vi "main.vi"() -> ()   [LabVIEW 2021]
uses:
  <vilib>/Analysis/Matrix/Datatypes/RealMatrix.ctl
  <vilib>/myRIO/Common/Instrument Driver Framework/myRIO v1.0/IRQ/typedefs/DI IRQ Type.ctl
  <vilib>/userDefined/High Color/nirio_resource_hc.ctl
  <vilib>/myRIO/Instrument Drivers/Onboard IO/PWM/typedefs/PWM Reference.ctl
  <vilib>/myRIO/Common/Instrument Driver Framework/Utilities/typedefs/myRIO Generic Hardware Reference.ctl
  <vilib>/myRIO/Common/Instrument Driver Framework/Utilities/typedefs/Hardware Version Enum.ctl
  <vilib>/myRIO/Common/Instrument Driver Framework/Utilities/typedefs/myRIO v1.0 Reference.ctl
  <vilib>/myRIO/Common/Instrument Driver Framework/Utilities/typedefs/Generic FPGA Reference.ctl
  <vilib>/myRIO/Common/Instrument Driver Framework/myRIO v1.0/PWM/typedefs/PWM Channels Enum.ctl
  <vilib>/myRIO/Instrument Drivers/Onboard IO/PWM/typedefs/PWM Configuration.ctl
  <vilib>/Platform/TimedLoop/XDataNode/timing_clust.ctl
  <vilib>/Platform/TimedLoop/XDataNode/nitl_modes.ctl
  <vilib>/Platform/TimedLoop/XDataNode/wakeup.ctl
  <vilib>/myRIO/Instrument Drivers/Onboard IO/PWM/vis/Set Duty Cycle and Frequency.vi
  ISRglobals.vi
  ISR.vi
  <vilib>/myRIO/Common/Instrument Driver Framework/myRIO v1.0/IRQ/vis/myRIO v1.1 Register DI IRQ.vi
  <vilib>/Analysis/Matrix/Numeric/Multiply/Multiply - RM,R.vi
  <vilib>/Analysis/Matrix/Numeric/Multiply/Multiply - RM,RM.vi
  <vilib>/myRIO/Common/Instrument Driver Framework/myRIO v1.0/PWM/vis/myRIO v1.0 Write PWM.vi
  <vilib>/myRIO/Express VI/IRQ/IRQ Express VI.xnode
  <vilib>/myRIO/Instrument Drivers/IRQ/IO IRQ/vis/myRIO Register DI IRQ.xnode
  <vilib>/myRIO/Common/Instrument Driver Framework/myRIO v1.0/IRQ/typedefs/Callback VI Ref.ctl
  <vilib>/platform/TimedLoop/XDataNode/XDataNode.xnode
  <vilib>/Platform/TimedLoop/XDataNode/XDNodeRunTimeDep.lvlib
  <vilib>/myRIO/Instrument Drivers/Onboard IO/PWM/PWM.lvlib
  <vilib>/Analysis/Matrix/NI_Matrix.lvlib
  <vilib>/ptbypt/NI_PtbyPt.lvlib
panel:
  out "theta RLS":dbl[][](graph)
  out "theta_RLS_1":dbl[](graph)
  out "theta_RLS_0":dbl[](graph)
  out "theta_RLS_2":dbl[](graph)
  out "theta_RLS_3":dbl[](graph)
  out "theta 3":dbl[](graph)
  out "theta 2":dbl[](graph)
  out "theta 1":dbl[](graph)
  out "theta 0":dbl[](graph)
  out "u":dbl
  out "PWM":dbl
  out "up":dbl
  out "uw":dbl
  out "Omega_d":dbl[][](graph)
  out "theta":dbl[][](graph)
  out "U":dbl[][](graph)
  out "th_max":T1
  out "th_min":T1
  out "th":T1
  out "T":dbl
  out "M":dbl
  out "N":i32
  out "i":i32
  out "Max. Iteration Duration":i64
  out "error out (no error) 2":errorcluster
  out "Iteration Duration":i64
  out "Interrupt On":bool
  out "Omega":dbl[][](graph)
  in  "error in (no error)":errorcluster
  out "Np":dbl
  out "ft":dbl
  out "Finished late":bool
  out "Run Time (s)":dbl=50.0
  out "Sampling \nFrequency (Hz)":dbl=250.0
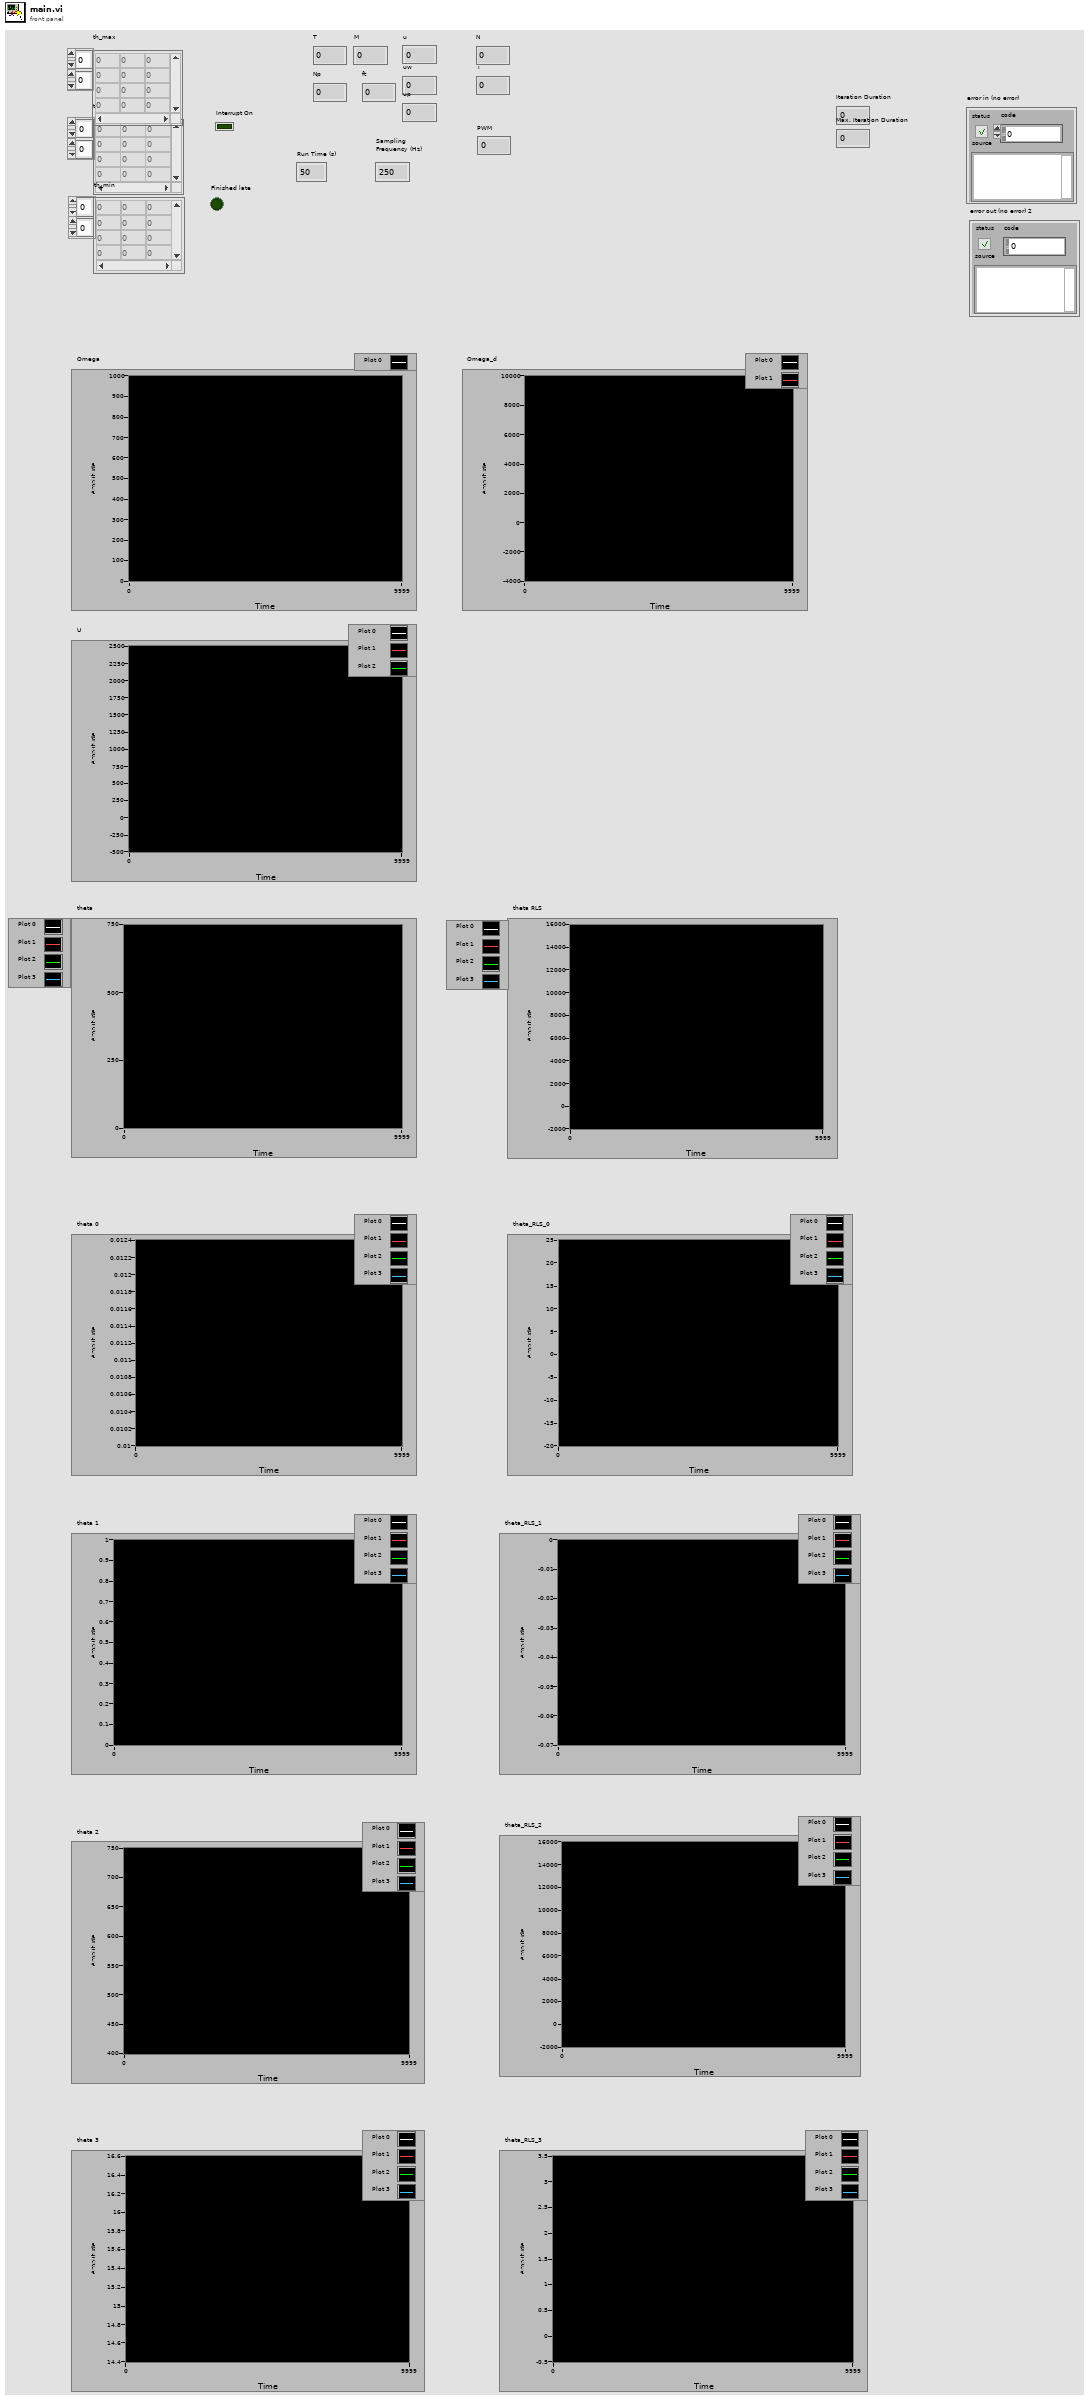
[diagram p1: front panel]
types:
  T1 = typedef "NI_Matrix.lvlib/RealMatrix.ctl" = dbl[][]
  T2 = typedef "DI IRQ Type.ctl" = enum16{"Digital falling edge", "Digital rising edge", "Digital edge"}
  T3 = typedef "nirio_resource_hc.ctl" = tag
  T4 = typedef "PWM.lvlib/PWM Reference.ctl" = cluster{"myRIO Reference":T5, "PWM Channels Enum":T9, "PWM Configuration":T10}
  T5 = typedef "myRIO Generic Hardware Reference.ctl" = cluster{"myRIO Model":T6, "myRIO Hardware Reference":T7}
  T6 = typedef "Hardware Version Enum.ctl" = enum16{"Unknown", "myRIO-1900", "myRIO-1950", "roboRIO", "NI ELVIS RIO CM", "ELVIS III"}
  T7 = typedef "myRIO v1.0 Reference.ctl" = cluster{"Generic FPGA Reference":T8, "Allow multiple opens":bool}
  T8 = typedef "Generic FPGA Reference.ctl" = refnum<k20>
  T9 = typedef "PWM Channels Enum.ctl" = enum16{"Not Connected", "C/PWM0", "C/PWM1", "A/PWM0", "A/PWM1", "A/PWM2", "A/PWM3", "A/PWM4", "A/PWM5", "A/PWM6", "A/PWM7", "A/PWM8", "A/PWM9", "A/PWM10", "A/PWM11", "A/PWM12", "A/PWM13", "A/PWM14", "A/PWM15", "A/PWM16", "A/PWM17", "A/PWM18", "A/PWM19", "B/PWM0", "B/PWM1", "B/PWM2", "B/PWM3", "B/PWM4", "B/PWM5", "B/PWM6", "B/PWM7", "B/PWM8", "B/PWM9", "B/PWM10", "B/PWM11", "B/PWM12", "B/PWM13", "B/PWM14", "B/PWM15", "B/PWM16", "B/PWM17", "B/PWM18", "B/PWM19", "PWM/PWM0", "PWM/PWM1", "PWM/PWM2", "PWM/PWM3", "PWM/PWM4", "PWM/PWM5", "PWM/PWM6", "PWM/PWM7", "PWM/PWM8", "PWM/PWM9"}
  T10 = typedef "PWM.lvlib/PWM Configuration.ctl" = cluster{"Frequency":dbl, "Duty Cycle":dbl}
  T11 = typedef "XDNodeRunTimeDep.lvlib/timing_clust.ctl" = cluster{"Expected End [f-1]":u64, "Actual End [f-1]":u64, "Finished Late? [f-1]":bool, "Expected End [i-1]":u64, "Actual End [i-1]":u64, "Finished Late? [i-1]":bool, "Expected Start [i]":u64, "Actual Start [i]":u64, "Expected Start [f]":u64, "Actual Start [f]":u64, "Source Name":string, "Structure Name":string, "Period":i64, "Deadline":i64, "Offset":i64, "Start":i64, "Priority":i32, "Timeout":i32, "Mode":T12, "Wakeup Reason":T13, "Error":errorcluster, "Source Type":string, "Secondary Source Type":string, "Global End Time":u64, "Global Start Time":u64, "Frame Duration":u64, "Iteration Duration":u64, "Assigned CPU":i32, "I/O Scan Engine Mode":u32}
  T12 = typedef "XDNodeRunTimeDep.lvlib/nitl_modes.ctl" = enum32{"No Change", "Process missed periods, maintain original phase", "Discard missed periods, maintain original phase", "Process missed periods, ignore original phase", "Discard missed periods, ignore original phase"}
  T13 = typedef "XDNodeRunTimeDep.lvlib/wakeup.ctl" = enum32{"Normal", "Aborted", "Asynchronous wakeup", "Timing source error", "Timed loop error", "Timeout"}
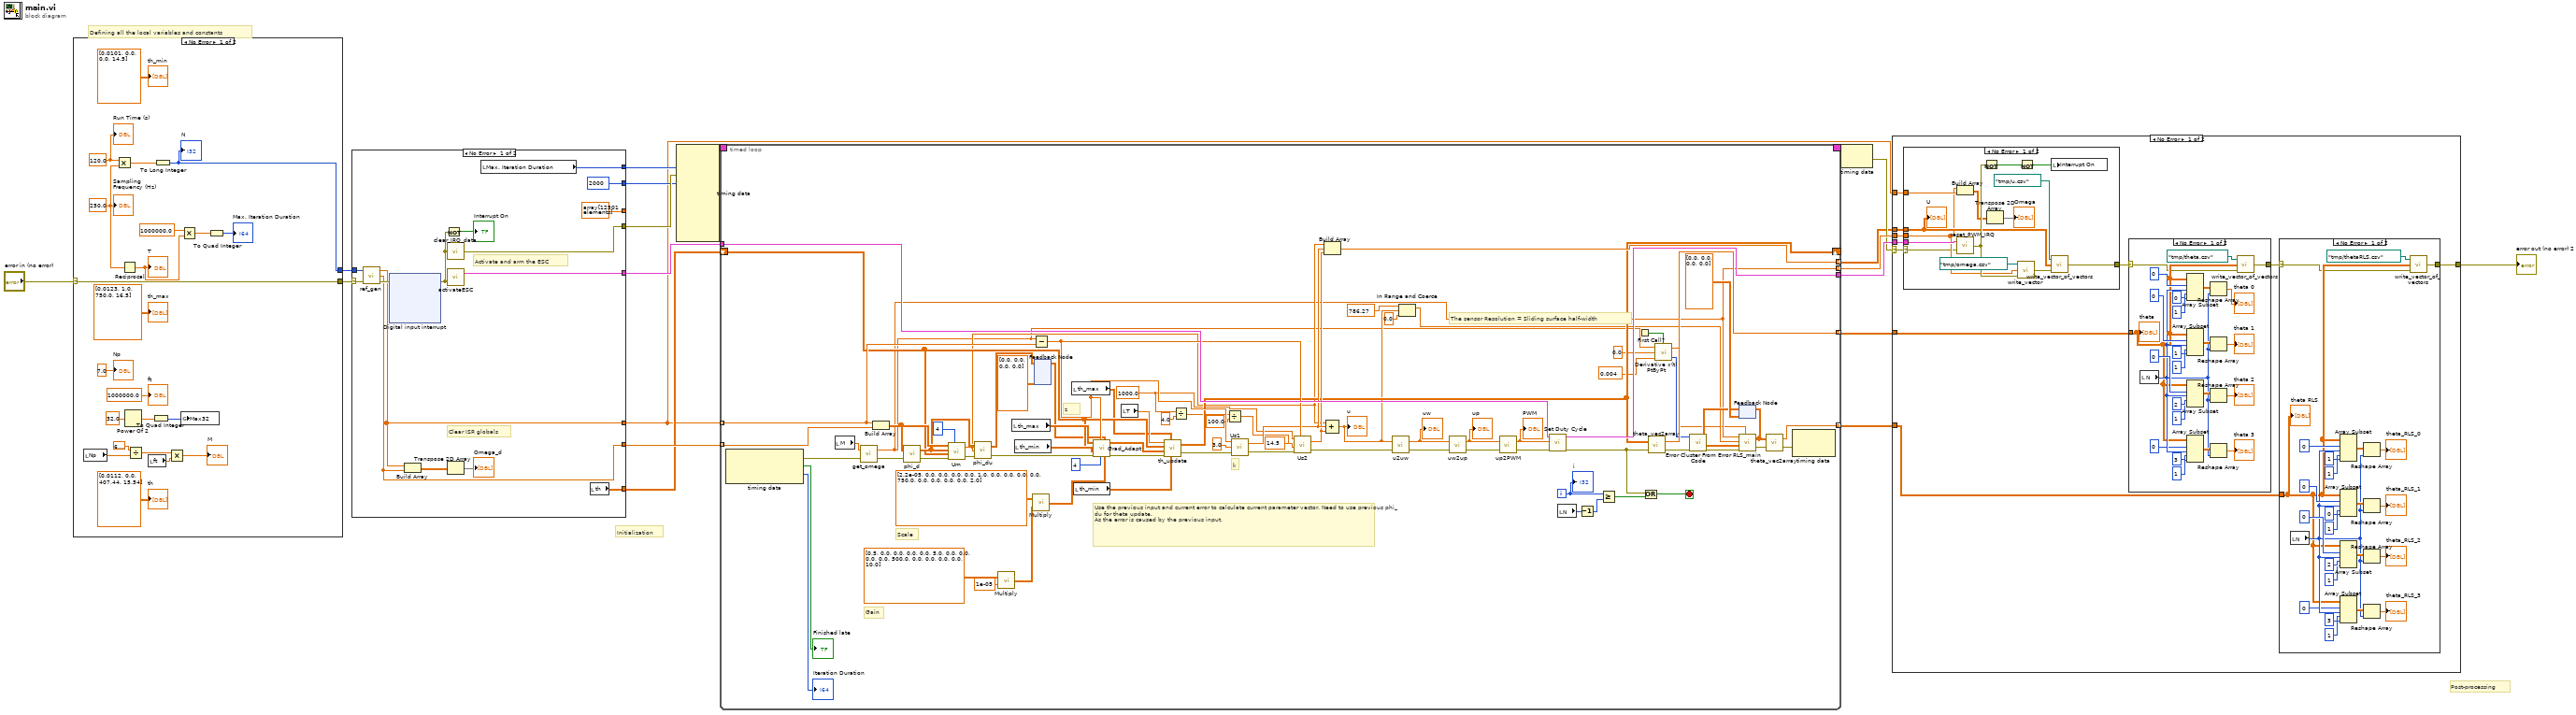
[diagram p0: block diagram]
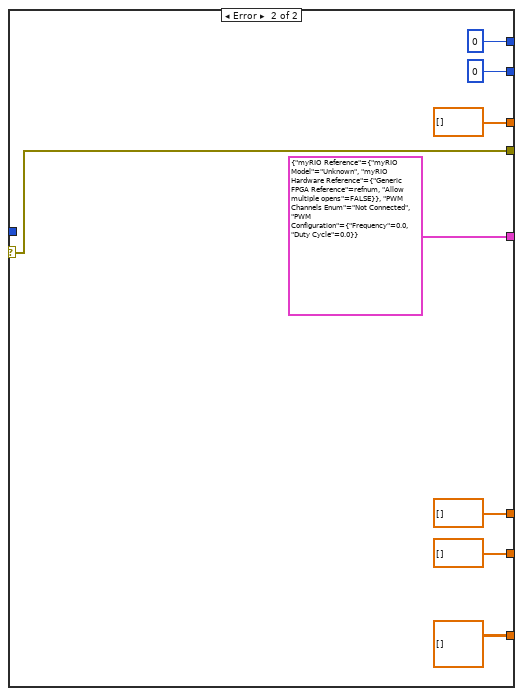
[diagram p2: hidden frame]
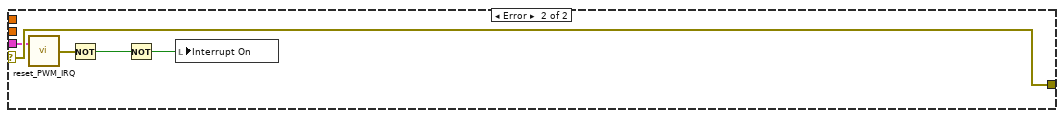
[diagram p6: hidden frame]
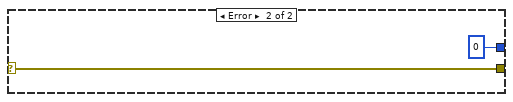
[diagram p7: hidden frame]
diagram:
  # "Post-processing"
  # "Initialization"
  # "Defining all the local variables and constants"
  n1 = case shown="No Error" "error in (no error)" {
    selector: "error in (no error)" -> [w39 w43]
    tunnel: [w39 w43] -> w15
    tunnel: [w25 0] -> w14
    frame No Error {
      w20 = 120.0 ("Run Time (s)")
      w21 = 250.0 ("Sampling \nFrequency (Hz)")
      n2 = local read "Np"() -> (w35:dbl)
      n3 = Multiply(x=w20, y=w21) -> (x*y=w28:dbl)
      n4 = Reciprocal(x=w21) -> (1/x=w31:dbl)
      "T" <- w31
      n5 = Power Of 2(x=32.0) -> (2^x=w41:dbl)
      n6 = Divide(x=6.283185307179586, y=w35) -> (x/y=w34:dbl)
      n7 = local read "ft"() -> (w33:dbl)
      n8 = To Quad Integer(1:w41) -> (0:w32:i64)
      n9 = To Long Integer(number=w28) -> (32bit integer=w25:i32)
      "N" <- w25
      n10 = Multiply(x=w34, y=w33) -> (x*y=→"M":dbl)
      n11 = Multiply(x=1000000.0, y=w31) -> (x*y=w30:dbl)
      n12 = global write "ISRglobals.vi" "Max32"(w32) -> ()
      n13 = To Quad Integer(1:w30) -> (0:→"Max. Iteration Duration":i64)
      "Np" <- 7.0 ("Numeric")
      "ft" <- 1000000.0 ("ft")
      "Run Time (s)" <- w20
      "Sampling \nFrequency (Hz)" <- w21
      "th_min" <- T1 [[0.0101], [0.0], [0.0], [14.5]] ("th")
      "th" <- T1 [[0.0112], [0.0], [407.44], [15.54]] ("th")
      "th_max" <- T1 [[0.0123], [1.0], [750.0], [16.5]] ("th")
    }
    frame Error {
    }
  }
  n14 = case shown="No Error" w15 {
    selector: w15 -> [w57 w83]
    tunnel: w14 -> [w58 _]
    tunnel: [w46 dbl[] [] ("xd")] -> w13
    tunnel: [w47 dbl[] [] ("x")] -> w2
    tunnel: [w54 w83] -> w12
    tunnel: [dbl[] array[12501 elements] dbl[] []] -> _
    tunnel: [2000 ("Priority") 0 ("Priority")] -> w11
    tunnel: [w50 i64 0 ("Max. Iteration Duration")] -> w10
    tunnel: [w49 T4 {"myRIO Reference"={"myRIO Model"=enum."Unknown", "myRIO Hardware Reference"={"Generic FPGA Reference"=refnum, "Allow multiple opens"=FALSE}}, "PWM Channels Enum"=enum."Not Connected", "PWM Configuration"={"Frequency"=0.0, "Duty Cycle"=0.0}} ("PWM Ref Out")] -> w9
    tunnel: [w48 T1 [] ("th")] -> w8
    frame No Error {
      # "Activate and arm the ESC"
      # "Clear ISR globals"
      n15 = call "ref_gen.vi"("error in (no error)"=w57, "N"=w58) -> ("error out"=w56:errorcluster, "xd"=w46:dbl[], "x"=w47:dbl[])  [unwired: 1 in]
      n16 = xnode "Digital input interrupt"("error in (no error)"=w56) -> ("error out"=w53:errorcluster)
      n17 = Build Array(w47, w46) -> (w45:dbl[][])
      n18 = Not(x=w53) -> (.not. x?=→"Interrupt On":bool)
      n19 = call "clear_IRQ_data.vi"("error IO"=w53) -> ("error IO 2"=w54:errorcluster)
      n20 = call "activateESC.vi"("error in (no error)"=w53) -> ("PWM Ref Out"=w49:T4)  [unwired: 1 in, 1 out]
      n21 = Transpose 2D Array(2D array=w45) -> (transposed array=→"Omega_d":dbl[][])
      n22 = local read "Max. Iteration Duration"() -> (w50:i64)
      n23 = local read "th"() -> (w48:T1)
    }
    frame Error {
    }
  }
  n24 = node-c288(w10, w12, w11) -> (w19:T11)  [unwired: 7 in]
  n25 = timed-loop {
    timing: w19 -> [_]
    timing-out: [_] -> w18
    tunnel: w9 -> [w162]
    tunnel: [w159] -> w6
    tunnel: w2 -> [w144] mode=indexing
    tunnel: w13 -> [w151] mode=indexing
    shift-right: [w120] -> _
    shift-left: w8 -> [w122]
    tunnel: [w89] -> w7 mode=indexing
    tunnel: [w127] -> w4 mode=indexing
    tunnel: [w125] -> w3 mode=indexing
    tunnel: [w96] -> w1 mode=indexing
    i -> [w157]
    stop <- w161 stop-if-true
    w112 = 1000.0 ("h")
    # "Use the previous input and current error to calculate current parameter vector. Need to use previous phi_du for theta update.\nAs the error is caused by the previous input."
    # "The sensor Resolution = Sliding surface half-width"
    # "Scale"
    # "Gain"
    # "k"
    # "z"
    n26 = node-c288() -> (w153:errorcluster, →"Finished late":bool, →"Iteration Duration":i64)  [unwired: 1 in]
    n27 = local read "M"() -> (w154:dbl)
    n28 = call "get_omega.vi"("error in (no error)"=w153, "M"=w154) -> ("error out"=w134:errorcluster, "omega"=w89:dbl)
    n29 = Build Array(w144, w151) -> (w150:T1)
    n30 = call "phi_d.vi"("error in (no error)"=w134, "x_d"=w150) -> ("error out"=w133:errorcluster, "phi_d"=w149:T1)
    n31 = call "Um.vi"("x_d"=w150, "phi_d"=w149, "theta"=w122, "error in (no error)"=w133, "N"=4) -> ("Um"=w107:dbl, "error out"=w106:errorcluster)
    n32 = call "phi_du.vi"("error in (no error)"=w106, "u_m"=w107, "phi_d"=w149) -> ("error out"=w132:errorcluster, "phi_du"=w104:T1)
    n33 = call-poly <vilib>:"Multiply.vi"("Real Scalar c"=1e-05, "Real Matrix A"=T1 [[0.5, 0.0, 0.0, 0.0], [0.0, 5.0, 0.0, 0.0], [0.0, 0.0, 500.0, 0.0], [0.0, 0.0, 0.0, 10.0]] ("Real Matrix B")) -> ("A * c"=w114:T1)
    n34 = local read "th_max"() -> (w147:T1)
    n35 = local read "th_min"() -> (w146:T1)
    n36 = call-poly <vilib>:"Multiply.vi"("Real Matrix B"=w114, "Real Matrix A"=T1 [[2.2e-05, 0.0, 0.0, 0.0], [0.0, 1.0, 0.0, 0.0], [0.0, 0.0, 750.0, 0.0], [0.0, 0.0, 0.0, 2.0]] ("Gamma")) -> ("A * B"=w105:T1)
    n37 = Subtract(x=w89, y=w144) -> (x-y=w141:dbl)
    n38 = feedback #1(T1 [[0.0], [0.0], [0.0], [0.0]] ("phi_du")) -> (w103:T1)
    n39 = feedback-in #1(w104) -> ()
    n40 = local read "th_max"() -> (w117:T1)
    n41 = local read "th_min"() -> (w118:T1)
    n42 = call "Grad_Adapt.vi"("Gamma"=w105, "phi_du"=w103, "N"=4, "z"=w141, "error in (no error)"=w132, "th_min"=w146, "th"=w122, "th_max"=w147) -> ("error out"=w121:errorcluster, "theta_dot"=w123:T1)  [unwired: 2 in]
    n43 = local read "T"() -> (w124:dbl)
    n44 = call "th_update.vi"("th_min"=w118, "th_max"=w117, "error in (no error)"=w121, "th_d"=w123, "th[k]"=w122, "dt"=w124) -> ("error out"=w119:errorcluster, "th[k+1]"=w120:T1)
    n45 = Divide(x=w112, y=4.0) -> (x/y=w110:dbl)
    n46 = Divide(x=w110, y=100.0) -> (x/y=w108:dbl)
    n47 = call "Us1.vi"("error in (no error)"=w119, "k"=3.0, "z"=w141) -> ("error out"=w131:errorcluster, "Us1"=w129:dbl)
    n48 = call "Us2.vi"("h"=w112, "eps"=w108, "\\hat b_min"=14.5 ("\\hat b_min"), "error in (no error)"=w131, "z"=w141) -> ("Us2"=w128:dbl, "error out"=w130:errorcluster)
    n49 = Build Array(w107, w129, w128) -> (w127:dbl[])
    n50 = Compound Arithmetic op=ADD(w107, w129, w128) -> (w99:dbl)
    "u" <- w99
    n51 = call "u2uw.vi"("error in (no error)"=w130, "u"=w99) -> ("error out"=w135:errorcluster, "uw"=w140:dbl)
    "uw" <- w140
    n52 = In Range and Coerce(upper limit=786.27, x=w99, lower limit=0.0) -> (coerced(x)=w92:dbl)  [unwired: 1 out]
    n53 = call "uw2up.vi"("error in (no error)"=w135, "uw"=w140) -> ("error out"=w136:errorcluster, "up"=w139:dbl)
    "up" <- w139
    n54 = call "up2PWM.vi"("error in (no error)"=w136, "up"=w139) -> ("error out"=w137:errorcluster, "PWM"=w138:dbl)
    "PWM" <- w138
    n55 = call <vilib>:"Set Duty Cycle.vi"("error in (no error)"=w137, "Duty Cycle"=w138, "PWM Ref In"=w162) -> ("error out"=w126:errorcluster, "PWM Ref Out"=w159:T4)  [unwired: 6 in]
    n56 = local read "N"() -> (w152:i32)
    n57 = Decrement(x=w152) -> (x-1=w158:i32)
    n58 = Greater Or Equal?(x=w157, y=w158) -> (x >= y?=w160:bool)
    n59 = First Call?() -> (First Call?: T/F=w87:bool)
    n60 = Or(x=w126, y=w160) -> (x .or. y?=w161:bool)
    n61 = call "theta_vec2array.vi"("error in (no error)"=w126, "Real Matrix"=w120) -> ("error out"=w85:errorcluster, "appended array"=w125:dbl[])
    n62 = call <vilib>:"Derivative x(t) PtByPt.vi"("initialize"=w87, "dt"=0.004, "initial condition"=0.0, "x"=w89) -> ("error"=w86:i32, "dx/dt"=w88:dbl)
    n63 = call <vilib>:"Error Cluster From Error Code.vi"("error in (no error)"=w85, "error code (0)"=w86) -> ("error out"=w84:errorcluster)  [unwired: 7 in]
    n64 = feedback #2(T1 [[0.0], [0.0], [0.0], [0.0]] ("\\theta (t)")) -> (w93:T1)
    n65 = call "RLS_main.vi"("dx/dt"=w88, "error in (no error)"=w84, "\\theta (t-1)"=w93, "u(t)"=w92, "x(t)"=w89) -> ("error out"=w95:errorcluster, "\\theta (t)"=w94:T1)  [unwired: 1 in]
    n66 = feedback-in #2(w94) -> ()
    n67 = call "theta_vec2array.vi"("error in (no error)"=w95, "Real Matrix"=w94) -> ("error out"=w97:errorcluster, "appended array"=w96:dbl[])
    n68 = node-c288(w97) -> ()  [unwired: 1 in, 1 out]
    "i" <- w157
  }
  n69 = node-c288(w18) -> (w5:errorcluster)
  n70 = case shown="No Error" w5 {
    selector: w5 -> [w174 w251]
    tunnel: [w170 w251] -> w16
    tunnel: w7 -> [w175 _]
    tunnel: w6 -> [w179 w250]
    tunnel: w4 -> [w178 _]
    tunnel: w3 -> [w176 _]
    tunnel: w2 -> [w177 _]
    tunnel: w1 -> [w172 _]
    frame No Error {
      n71 = case shown="No Error" w174 {
        selector: w174 -> [w233 w246]
        tunnel: w179 -> [w245 _]
        tunnel: w178 -> [w239 _]
        tunnel: w177 -> [w237 _]
        tunnel: w175 -> [w234 _]
        tunnel: [w232 w246] -> w173
        frame No Error {
          n72 = Build Array(w234, w237) -> (w236:dbl[][])
          n73 = call "reset_PWM_IRQ.vi"("error in (no error)"=w233, "PWM Ref In"=w245) -> ("error out"=w242:errorcluster)
          n74 = Not(x=w242) -> (.not. x?=w243:bool)
          n75 = Transpose 2D Array(2D array=w236) -> (transposed array=→"Omega":dbl[][])
          n76 = call "write_vector.vi"("error in (no error)"=w242, "1D data"=w234, "file path (dialog if empty)"=path "/tmp/omega.csv" ("RPM Inst Data")) -> ("error out"=w241:errorcluster)
          n77 = Not(x=w243) -> (.not. x?=w244:bool)
          n78 = local write "Interrupt On"(w244) -> ()
          n79 = call "write_vector_of_vectors.vi"("error in (no error)"=w241, "2D data"=w239, "file path (dialog if empty)"=path "/tmp/u.csv") -> ("error out"=w232:errorcluster)
          "U" <- w239
        }
        frame Error {
        }
      }
      n80 = case shown="No Error" w173 {
        selector: w173 -> [w207 w231]
        tunnel: w176 -> [w208 _]
        tunnel: [w206 w231] -> w171
        frame No Error {
          n81 = local read "N"() -> (w210:i32)
          n82 = Array Subset(array=w208, index (row)=0 ("index"), length (row)=w210, index (col)=0 ("index"), length (col)=1 ("length")) -> (w222:dbl[][])
          n83 = Array Subset(array=w208, index (row)=0 ("index"), length (row)=w210, index (col)=1 ("index"), length (col)=1 ("length")) -> (w223:dbl[][])
          n84 = Array Subset(array=w208, index (row)=0 ("index"), length (row)=w210, index (col)=2 ("index"), length (col)=1 ("length")) -> (w219:dbl[][])
          n85 = Array Subset(array=w208, index (row)=0 ("index"), length (row)=w210, index (col)=3 ("index"), length (col)=1 ("length")) -> (w214:dbl[][])
          n86 = Reshape Array(w222, w210) -> (→"theta 0":dbl[])
          n87 = Reshape Array(w223, w210) -> (→"theta 1":dbl[])
          n88 = Reshape Array(w219, w210) -> (→"theta 2":dbl[])
          n89 = Reshape Array(w214, w210) -> (→"theta 3":dbl[])
          n90 = call "write_vector_of_vectors.vi"("error in (no error)"=w207, "2D data"=w208, "file path (dialog if empty)"=path "/tmp/theta.csv") -> ("error out"=w206:errorcluster)
          "theta" <- w208
        }
        frame Error {
        }
      }
      n91 = case shown="No Error" w171 {
        selector: w171 -> [w181 w205]
        tunnel: w172 -> [w182 _]
        tunnel: [w180 w205] -> w170
        frame No Error {
          n92 = local read "N"() -> (w184:i32)
          n93 = Array Subset(array=w182, index (row)=0 ("index"), length (row)=w184, index (col)=1 ("index"), length (col)=1 ("length")) -> (w197:dbl[][])
          n94 = Array Subset(array=w182, index (row)=0 ("index"), length (row)=w184, index (col)=0 ("index"), length (col)=1 ("length")) -> (w196:dbl[][])
          n95 = Array Subset(array=w182, index (row)=0 ("index"), length (row)=w184, index (col)=2 ("index"), length (col)=1 ("length")) -> (w193:dbl[][])
          n96 = Array Subset(array=w182, index (row)=0 ("index"), length (row)=w184, index (col)=3 ("index"), length (col)=1 ("length")) -> (w188:dbl[][])
          n97 = Reshape Array(w197, w184) -> (→"theta_RLS_0":dbl[])
          n98 = Reshape Array(w196, w184) -> (→"theta_RLS_1":dbl[])
          n99 = Reshape Array(w193, w184) -> (→"theta_RLS_2":dbl[])
          n100 = Reshape Array(w188, w184) -> (→"theta_RLS_3":dbl[])
          n101 = call "write_vector_of_vectors.vi"("error in (no error)"=w181, "2D data"=w182, "file path (dialog if empty)"=path "/tmp/thetaRLS.csv") -> ("error out"=w180:errorcluster)
          "theta RLS" <- w182
        }
        frame Error {
        }
      }
    }
    frame Error {
      n102 = call "reset_PWM_IRQ.vi"("PWM Ref In"=w250) -> ("error out"=w248:errorcluster)  [unwired: 1 in]
      n103 = Not(x=w248) -> (.not. x?=w249:bool)
      n104 = Not(x=w249) -> (.not. x?=w247:bool)
      n105 = local write "Interrupt On"(w247) -> ()
    }
  }
  "error out (no error) 2" <- w16
